vi "solar_cfg Flatten String to Variant.vi"(8 "error in (no error)":errorcluster, 9 "Keep Attributes? (F)":bool, 10 "Data String":string, 11 "Variant in":variant) -> (0 "error out":errorcluster, 1 "Valid?":bool, 3 "Variant out":variant)   [LabVIEW 2018]
doc: "This VI sets the variant value. This retains the attributes and type string."
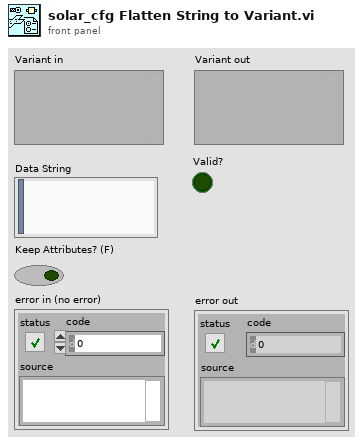
[diagram p1: front panel]
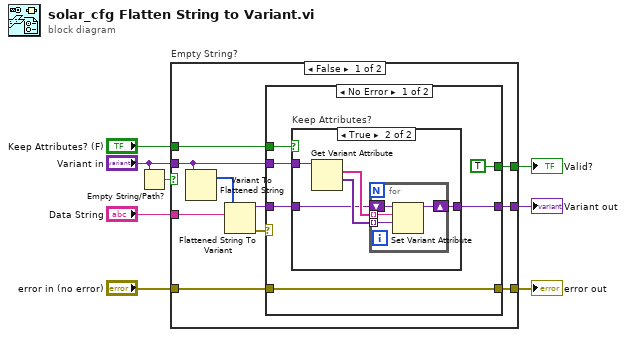
[diagram p0: block diagram]
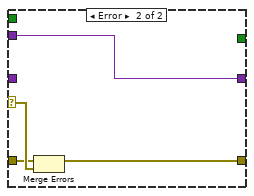
[diagram p3: hidden frame]
diagram:
  n1 = Empty String/Path?(string/path="Variant in") -> (empty?=w1:bool)
  n2 = case "Empty String?" shown="False" w1 {
    tunnel: "Variant in" -> [w16 w40]
    tunnel: "Data String" -> [w14 _]
    tunnel: [w13 _] -> w8
    tunnel: [w12 w40] -> w7
    tunnel: "Keep Attributes? (F)" -> [w11 _]
    tunnel: "error in (no error)" -> [w10 w39]
    tunnel: [w9 w39] -> w3
    frame False {
      n3 = Variant To Flattened String(Variant=w16) -> (1:w15:i16[])  [unwired: 1 out]
      n4 = Flattened String To Variant(6:w14, 7:w15) -> (0:w17:errorcluster, 3:w18:variant)  [unwired: 1 in]
      n5 = case shown="No Error" w17 {
        selector: w17 -> [_ w37]
        tunnel: [w24 w38] -> w12
        tunnel: w16 -> [w23 w38]
        tunnel: w18 -> [w22 _]
        tunnel: [TRUE _] -> w13
        tunnel: w11 -> [w20 _]
        tunnel: w10 -> [w19 w36]
        tunnel: [w19 w35] -> w9
        frame No Error {
          n6 = case "Keep Attributes?" shown="True" w20 {
            tunnel: [w25 w30] -> w24
            tunnel: w23 -> [_ w27]
            tunnel: w22 -> [w25 w26]
            frame False {
            }
            frame True {
              n7 = Get Variant Attribute(Variant=w27) -> (names=w29:string[], values=w28:variant[])  [unwired: 3 in, 2 out]
              n8 = for {
                tunnel: w29 -> [w33] mode=indexing
                tunnel: w28 -> [w32] mode=indexing
                shift-right: [w31] -> w30
                shift-left: w26 -> [w34]
                n9 = Set Variant Attribute(Variant=w34, name=w33, value=w32) -> (Variant out=w31:variant)  [unwired: 1 in, 2 out]
              }
            }
          }
        }
        frame Error {
          n10 = Merge Errors(w36, w37) -> (w35:errorcluster)
        }
      }
    }
    frame True {
    }
  }
  "Variant out" <- w7
  "Valid?" <- w8
  "error out" <- w3
